vi "Call By Invoke.vi"() -> ()   [LabVIEW 2020]
panel:
  in  "Item":i32(listbox)
  in  "Exit":bool
  # "运行的模块"
  # "选择模块"
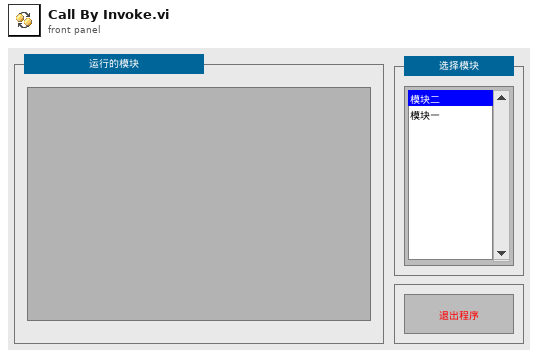
[diagram p1: front panel]
types:
  T1 = enum8{"Enabled", "Disabled", "Disabled and Grayed Out"}
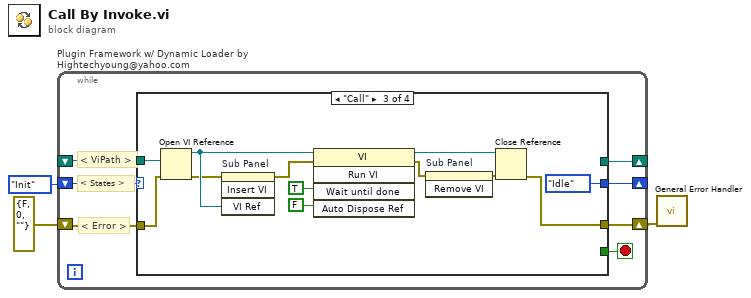
[diagram p0: block diagram]
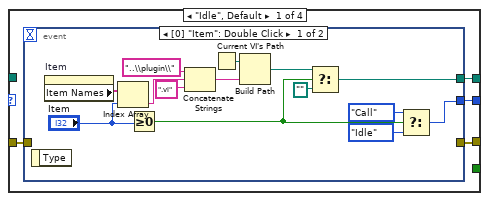
[diagram p2: hidden frame]
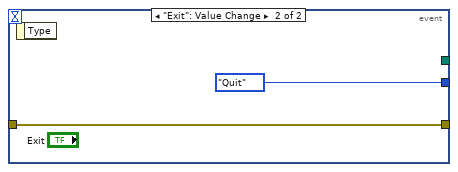
[diagram p3: hidden frame]
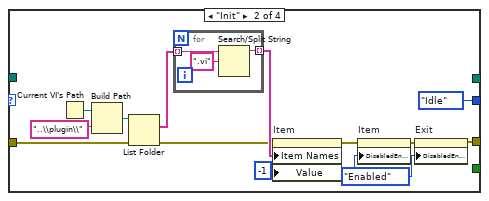
[diagram p4: hidden frame]
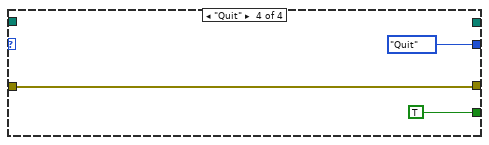
[diagram p5: hidden frame]
diagram:
  n1 = while "Plugin Framework w/ Dynamic Loader by Hightechyoung@yahoo.com" {
    shift-right: [w5] -> w3
    shift-left: errorcluster {"status"=FALSE, "code"=0, "source"=""} ("ErrorI") -> [w8]
    shift-right: [w9] -> _
    shift-left: enum16{"Idle", "Init", "Call", "Quit"}."Init" -> [w10]
    shift-right: [w6] -> _
    shift-left: _ -> [w4]
    stop <- w7 stop-if-true
    # "< Error >"
    # "< ViPath >"
    # "< States >"
    n2 = case shown="\"Call\"" w10 {
      tunnel: [w13 enum16{"Idle", "Init", "Call", "Quit"}."Idle" enum16{"Idle", "Init", "Call", "Quit"}."Idle" enum16{"Idle", "Init", "Call", "Quit"}."Quit"] -> w9
      tunnel: w8 -> [w14 w36 w55 w59]
      tunnel: [_ _ _ TRUE] -> w7
      tunnel: [w12 _ _ _] -> w6
      tunnel: [w11 w32 w50 w59] -> w5
      tunnel: w4 -> [_ _ w56 _]
      frame "Idle", Default {
        n3 = event shown="[0] \"Item\": Double Click" {
          selector: _ -> [_ _]
          dyn-events: _ -> [_ _]
          timeout: _ -> [_ _]
          tunnel: w14 -> [_ w29]
          tunnel: [w23 enum16{"Idle", "Init", "Call", "Quit"}."Quit"] -> w13
          tunnel: [w22 _] -> w12
          tunnel: [_ w29] -> w11
          event "Item": Double Click {
            n4 = event-data() -> ()  [unwired: 1 in, 1 out]
            n5 = property on="Item" class="LstBox (strict)"() -> ("Item Names"=w21:string[])  [unwired: 2 in, 2 out]
            n6 = Index Array(array=w21, index="Item") -> (element=w18:string)
            n7 = Greater Or Equal To 0?(x="Item") -> (x >= 0?=w26:bool)
            n8 = Concatenate Strings("..\\plugin\\" ("name or relative path"), w18, ".vi" ("string")) -> (w16:string)
            n9 = Current VI's Path() -> (path=w20:path)
            n10 = Build Path(base path=w20, name or relative path=w16) -> (appended path=w15:path)
            n11 = Select(t=w15, s=w26, f=path "") -> (s? t:f=w22:path)
            n12 = Select(t=enum16{"Idle", "Init", "Call", "Quit"}."Call", s=w26, f=enum16{"Idle", "Init", "Call", "Quit"}."Idle") -> (s? t:f=w23:enum16{"Idle", "Init", "Call", "Quit"})
          }
          event "Exit": Value Change {
            n13 = event-data() -> ()  [unwired: 1 in, 1 out]
          }
        }
      }
      frame "Init" {
        w31 = T1."Enabled" ("Disabled")
        n14 = Current VI's Path() -> (path=w40:path)
        n15 = Build Path(base path=w40, name or relative path="..\\plugin\\") -> (appended path=w39:path)
        n16 = List Folder(path=w39, error in=w36) -> (filenames=w37:string[], error out=w35:errorcluster)  [unwired: 2 in, 2 out]
        n17 = for {
          tunnel: w37 -> [w45] mode=indexing
          tunnel: [w44] -> w43 mode=indexing
          n18 = Search/Split String(string=w45, search string/char (-)=".vi" ("search string")) -> (substring before match=w44:string)  [unwired: 1 in, 2 out]
        }
        n19 = property on="Item" class="LstBox (strict)"(error in=w35, "Item Names"=w43, "Value"=-1 ("Item")) -> (error out=w33:errorcluster)  [unwired: 1 in, 1 out]
        n20 = property on="Item" class="LstBox (strict)"(error in=w33, "DisabledEnum"=w31) -> (error out=w34:errorcluster)  [unwired: 1 in, 1 out]
        n21 = property on="Exit" class="Bool"(error in=w34, "DisabledEnum"=w31) -> (error out=w32:errorcluster)  [unwired: 1 in, 1 out]
      }
      frame "Call" {
        n22 = Open VI Reference(vi path=w56, error in (no error)=w55) -> (vi reference=w54:refnum<vi>, error out=w53:errorcluster)  [unwired: 4 in]
        n23 = invoke on="Sub Panel" class="SubPnl" method="Insert VI"(error in=w53, "VI Ref"=w54) -> (error out=w52:errorcluster)  [unwired: 2 in, 3 out]
        n24 = invoke class="VI" method="Run VI"(reference=w54, error in=w52, "Wait until done"=TRUE ("结束前等待"), "Auto Dispose Ref"=FALSE ("Auto Dispose Reference")) -> (reference out=w48:refnum<vi>, error out=w49:errorcluster)  [unwired: 1 in, 3 out]
        n25 = invoke on="Sub Panel" class="SubPnl" method="Remove VI"(error in=w49) -> (error out=w51:errorcluster)  [unwired: 2 in, 2 out]
        n26 = Close Reference(reference=w48, error in (no error)=w51) -> (error out=w50:errorcluster)
      }
      frame "Quit" {
      }
    }
  }
  n27 = call <vilib>:"General Error Handler.vi"("error in (no error)"=w3) -> ()  [unwired: 10 in, 5 out]
